vi "LVAPT_Git_OnCommand(SingleObject).vi"(10 "Command ID":string, 11 "Object":T1) -> ()   [LabVIEW 2019]
uses:
  <resource>/Framework/Providers/API/ItemRef.ctl
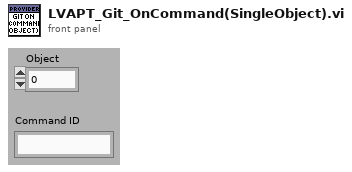
[diagram p1: front panel]
types:
  T1 = typedef "ItemRef.ctl" = u64
  T2 = enum16{"Action - None", "Action - RunPathInputVI"}
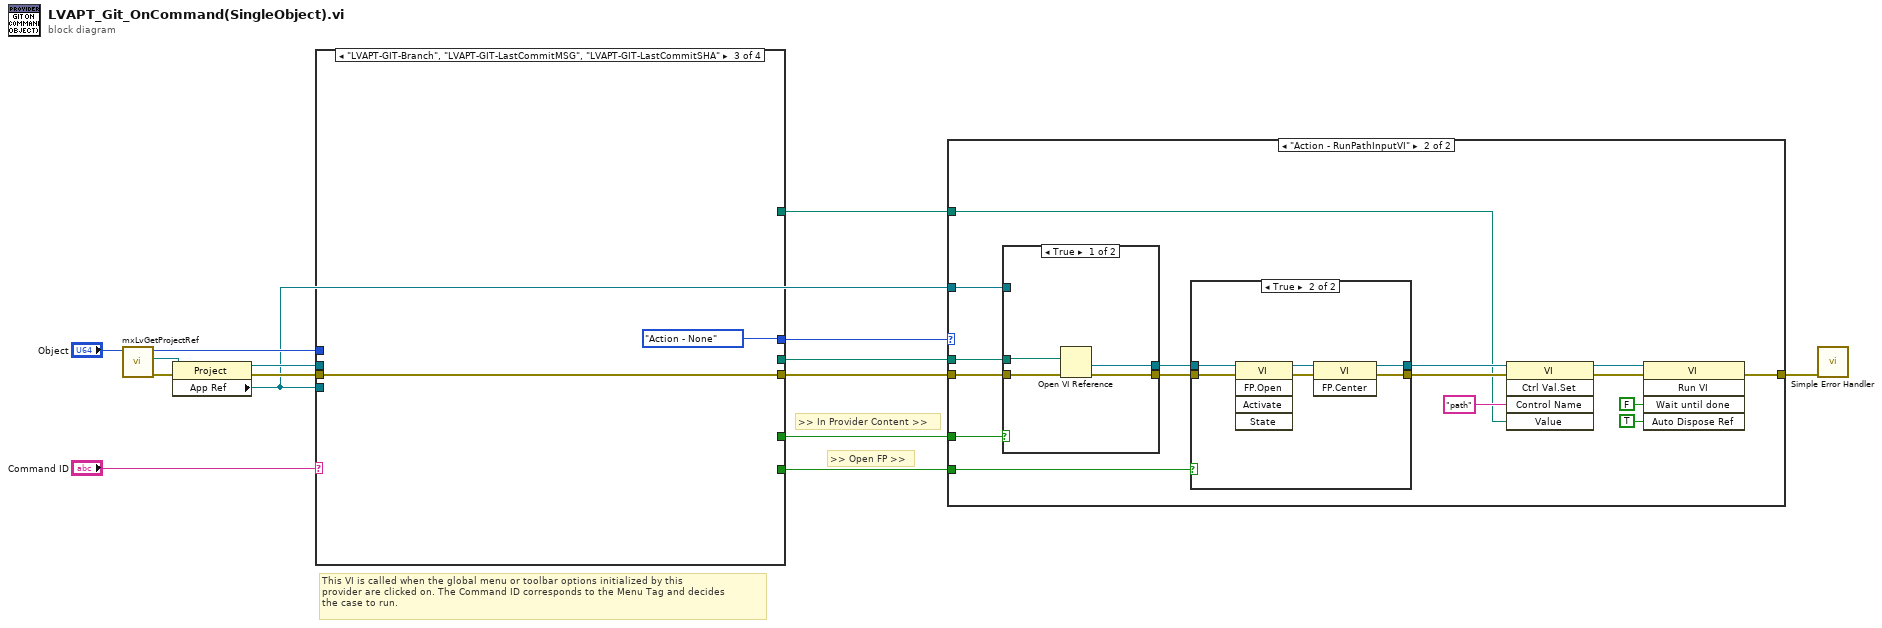
[diagram p0: block diagram]
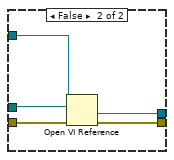
[diagram p4: hidden frame]
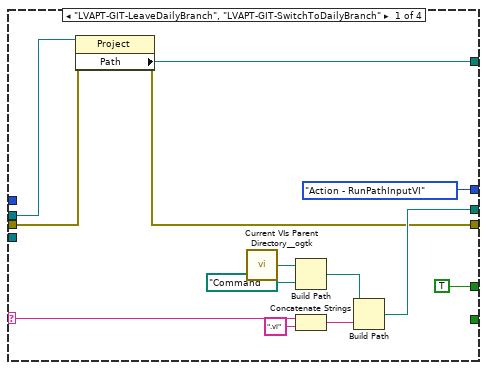
[diagram p5: hidden frame]
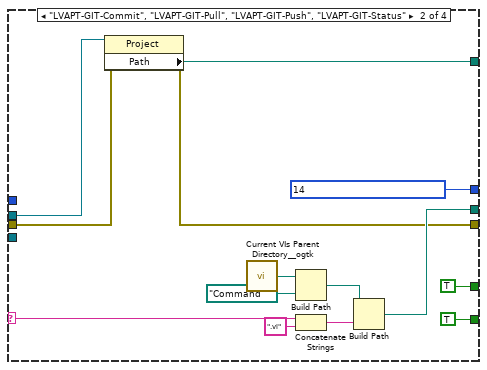
[diagram p6: hidden frame]
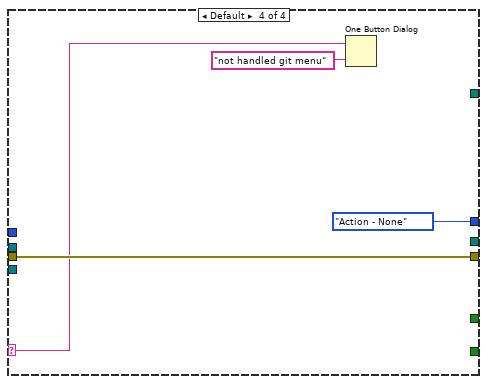
[diagram p7: hidden frame]
diagram:
  # ">> Open FP >>"
  # ">> In Provider Content >>"
  # "This VI is called when the global menu or toolbar options initialized by this \nprovider are clicked on. The Command ID corresponds to the Menu Tag and decides\nthe case to run."
  n1 = call <resource>:"mxLvGetProjectRef.vi"("Item"="Object") -> ("error out"=w14:errorcluster, "Project Refnum"=w13:refnum<vi>, "Item"=w11:T1)  [unwired: 8 in]
  n2 = property class="Project"(reference=w13, error in=w14) -> (reference out=w9:refnum<vi>, error out=w10:errorcluster, "App Ref"=w6:refnum<vi>)
  n3 = case shown="\"LVAPT-GIT-Branch\", \"LVAPT-GIT-LastCommitMSG\", \"LVAPT-GIT-LastCommitSHA\"" "Command ID" {
    selector: "Command ID" -> [w23 w35 _ w47]
    tunnel: [w18 w30 w44 w48] -> w5
    tunnel: w11 -> [_ _ _ _]
    tunnel: w10 -> [w19 w31 w44 w48]
    tunnel: w6 -> [_ _ _ _]
    tunnel: w9 -> [w20 w32 _ _]
    tunnel: [T2."Action - RunPathInputVI" T2 14 T2."Action - None" T2."Action - None"] -> w7
    tunnel: [w24 w36 _ _] -> w4
    tunnel: [_ TRUE _ _] -> w3
    tunnel: [TRUE TRUE _ _] -> w2
    tunnel: [w17 w29 _ _] -> w1
    frame "LVAPT-GIT-LeaveDailyBranch", "LVAPT-GIT-SwitchToDailyBranch" {
      n4 = property class="Project"(reference=w20, error in=w19) -> (error out=w18:errorcluster, "Path"=w17:path)  [unwired: 1 out]
      n5 = call <userlib>:"Current VIs Parent Directory__ogtk.vi"() -> ("Parent Directory (+ Relative)"=w28:path)  [unwired: 5 in]
      n6 = Build Path(base path=w28, name or relative path=path "Command") -> (appended path=w25:path)
      n7 = Concatenate Strings(w23, ".vi" ("string")) -> (w21:string)
      n8 = Build Path(base path=w25, name or relative path=w21) -> (appended path=w24:path)
    }
    frame "LVAPT-GIT-Commit", "LVAPT-GIT-Pull", "LVAPT-GIT-Push", "LVAPT-GIT-Status" {
      n9 = property class="Project"(reference=w32, error in=w31) -> (error out=w30:errorcluster, "Path"=w29:path)  [unwired: 1 out]
      n10 = call <userlib>:"Current VIs Parent Directory__ogtk.vi"() -> ("Parent Directory (+ Relative)"=w42:path)  [unwired: 5 in]
      n11 = Build Path(base path=w42, name or relative path=path "Command") -> (appended path=w37:path)
      n12 = Concatenate Strings(w35, ".vi" ("string")) -> (w33:string)
      n13 = Build Path(base path=w37, name or relative path=w33) -> (appended path=w36:path)
    }
    frame "LVAPT-GIT-Branch", "LVAPT-GIT-LastCommitMSG", "LVAPT-GIT-LastCommitSHA" {
    }
    frame Default {
      n14 = One Button Dialog(message=w47, button name ("OK")="not handled git menu") -> ()  [unwired: 1 out]
    }
  }
  n15 = case shown="\"Action - RunPathInputVI\"" w7 {
    tunnel: w5 -> [w49 w65]
    tunnel: w6 -> [_ w64]
    tunnel: [w49 w63] -> w8
    tunnel: w4 -> [_ w57]
    tunnel: w3 -> [_ w51]
    tunnel: w2 -> [_ w56]
    tunnel: w1 -> [_ w50]
    frame "Action - None", Default {
    }
    frame "Action - RunPathInputVI" {
      n16 = case shown="True" w56 {
        tunnel: w65 -> [w77 w82]
        tunnel: w64 -> [_ w81]
        tunnel: [w76 w80] -> w55
        tunnel: [w75 w79] -> w54
        tunnel: w57 -> [w74 w78]
        frame True {
          n17 = Open VI Reference(vi path=w74, error in (no error)=w77) -> (vi reference=w76:refnum<vi>, error out=w75:errorcluster)  [unwired: 4 in]
        }
        frame False {
          n18 = Open VI Reference(application reference (local)=w81, vi path=w78, error in (no error)=w82) -> (vi reference=w80:refnum<vi>, error out=w79:errorcluster)  [unwired: 3 in]
        }
      }
      n19 = case shown="True" w51 {
        tunnel: w55 -> [w67 w73]
        tunnel: [w67 w68] -> w52
        tunnel: [w66 w69] -> w53
        tunnel: w54 -> [w66 w72]
        frame False {
        }
        frame True {
          n20 = invoke class="VI" method="FP.Open"(reference=w73, error in=w72) -> (reference out=w71:refnum<vi>, error out=w70:errorcluster)  [unwired: 3 in, 3 out]
          n21 = invoke class="VI" method="FP.Center"(reference=w71, error in=w70) -> (reference out=w68:refnum<vi>, error out=w69:errorcluster)  [unwired: 1 in, 1 out]
        }
      }
      n22 = invoke class="VI" method="Ctrl Val.Set"(reference=w52, error in=w53, "Control Name"="path", "Value"=w50) -> (reference out=w59:refnum<vi>, error out=w58:errorcluster)  [unwired: 1 in, 3 out]
      n23 = invoke class="VI" method="Run VI"(reference=w59, error in=w58, "Wait until done"=FALSE ("Wait Until Done"), "Auto Dispose Ref"=TRUE ("Auto Dispose Reference")) -> (error out=w63:errorcluster)  [unwired: 1 in, 4 out]
    }
  }
  n24 = call <vilib>:"Simple Error Handler.vi"("error in (no error)"=w8) -> ()  [unwired: 4 in, 5 out]
